vi "TREE_open-close tree.vi"(8 "error in":errorcluster, 10 "Open/Close tree (F=CLOSE)":bool, 11 "Tree In":refnum<vi>) -> (0 "error out":errorcluster, 3 "Tree Out":refnum<vi>)   [LabVIEW 2011]
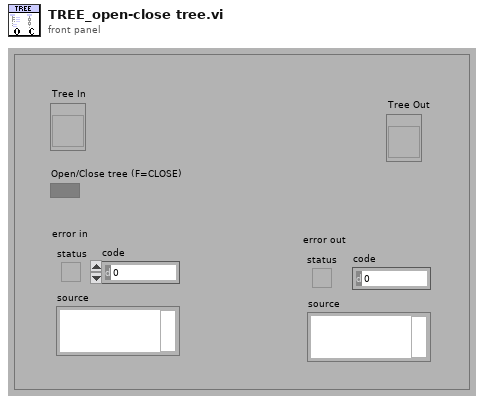
[diagram p1: front panel]
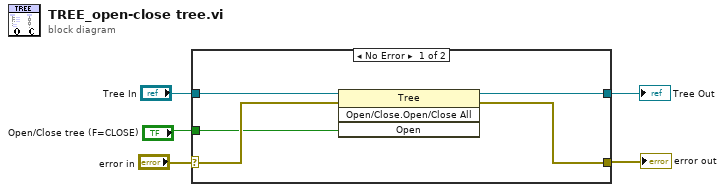
[diagram p0: block diagram]
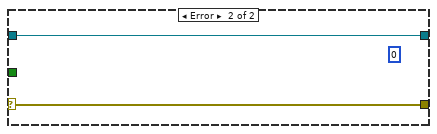
[diagram p2: hidden frame]
diagram:
  n1 = case shown="No Error" "error in" {
    selector: "error in" -> [w7 w12]
    tunnel: "Tree In" -> [w10 w11]
    tunnel: [w9 w11] -> w4
    tunnel: [w8 w12] -> w3
    tunnel: "Open/Close tree (F=CLOSE)" -> [w6 _]
    frame No Error {
      n2 = invoke on="Invoke Node" class="Tree" method="Open/Close.Open/Close All"(reference=w10, error in=w7, "Open"=w6) -> (reference out=w9:refnum<vi>, error out=w8:errorcluster)  [unwired: 1 in, 2 out]
    }
    frame Error {
      (unwired) 0 ("Number of files found")
    }
  }
  "Tree Out" <- w4
  "error out" <- w3
